vi "OutbitsClearMemory.vi"   [LabVIEW 2014]
uses:
  <vilib>/rvi/Emulation/niFpgaGetClockAttributes.vi
  <vilib>/rvi/Emulation/niFpgaSctlEmulationGetInTimedLoop.vi
  <vilib>/rvi/Emulation/niFpgaEmulationReportErrorSimple.vi
  <vilib>/rvi/Memory/Memory_Emulation/nirvimemoryFastEmulation.vi
  <vilib>/rvi/Memory/Memory_Emulation/nirvimemoryEmulation.vi
  <vilib>/rvi/Emulation/niFpgaEmulationIsFPGAContextNoSignature.vi
  <vilib>/rvi/DataTransferAndStorage/Container/Common/niFpgaContainerGetUniqueNameForEmu.vi
  <vilib>/rvi/Emulation/niFpgaProcessEmulError.vi
  <vilib>/rvi/errors/nirviReportUnexpectedCaseInternalError (U32).vi
  <vilib>/rvi/Emulation/niFpgaCriticalErrorInLSC.vi
  <vilib>/rvi/DataTransferAndStorage/Container/XNode/niFpgaContainer.xnode
panel:
  # "This will write zeros to all memory addresses"
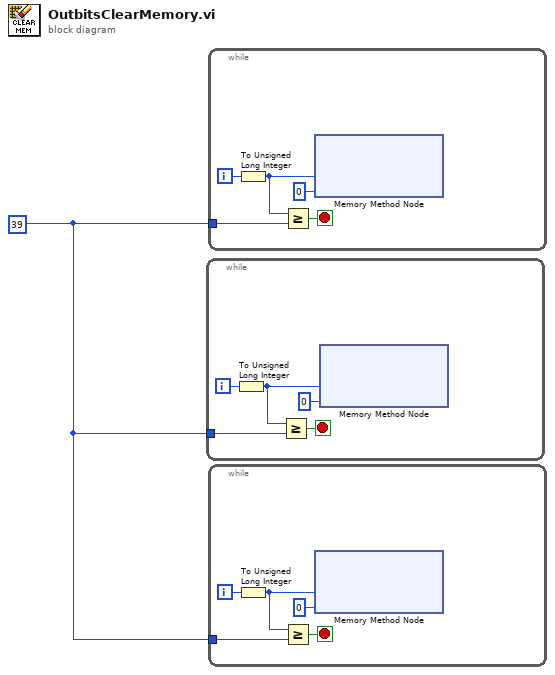
[diagram p0: block diagram]
diagram:
  w1 = u32 39
  n1 = while {
    tunnel: w1 -> [w5]
    i -> [w6]
    stop <- w4 stop-if-true
    n2 = To Unsigned Long Integer(number=w6) -> (unsigned 32bit integer=w3:u32)
    n3 = Greater Or Equal?(x=w3, y=w5) -> (x >= y?=w4:bool)
    n4 = xnode ("Memory Method Node")("Address"=w3, "Data"=u32 0) -> ()  [unwired: 1 in, 1 out]
  }
  n5 = while {
    tunnel: w1 -> [w9]
    i -> [w11]
    stop <- w8 stop-if-true
    n6 = To Unsigned Long Integer(number=w11) -> (unsigned 32bit integer=w10:u32)
    n7 = Greater Or Equal?(x=w10, y=w9) -> (x >= y?=w8:bool)
    n8 = xnode ("Memory Method Node")("Address"=w10, "Data"=u32 0) -> ()  [unwired: 1 in, 1 out]
  }
  n9 = while {
    tunnel: w1 -> [w15]
    i -> [w16]
    stop <- w14 stop-if-true
    n10 = To Unsigned Long Integer(number=w16) -> (unsigned 32bit integer=w13:u32)
    n11 = Greater Or Equal?(x=w13, y=w15) -> (x >= y?=w14:bool)
    n12 = xnode ("Memory Method Node")("Address"=w13, "Data"=u32 0) -> ()  [unwired: 1 in, 1 out]
  }
